vi "Find Best Merge Candidate.vi"(11 "Lines":T1[](array[typedef])) -> (0 "Best Match Outlier Distance":dbl, 2 "Best match second index":i32, 3 "Best match first index":i32)   [LabVIEW 2017]
uses:
  Vector Library/Line.ctl
  Vector Library/Vector.ctl
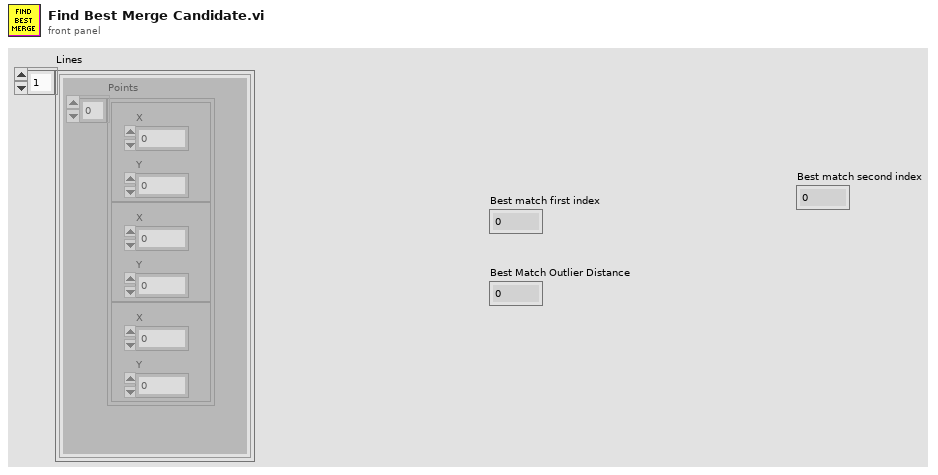
[diagram p1: front panel]
types:
  T1 = typedef "Line.ctl" = cluster{"Points":T2[]}
  T2 = typedef "Vector.ctl" = cluster{"X":dbl, "Y":dbl}
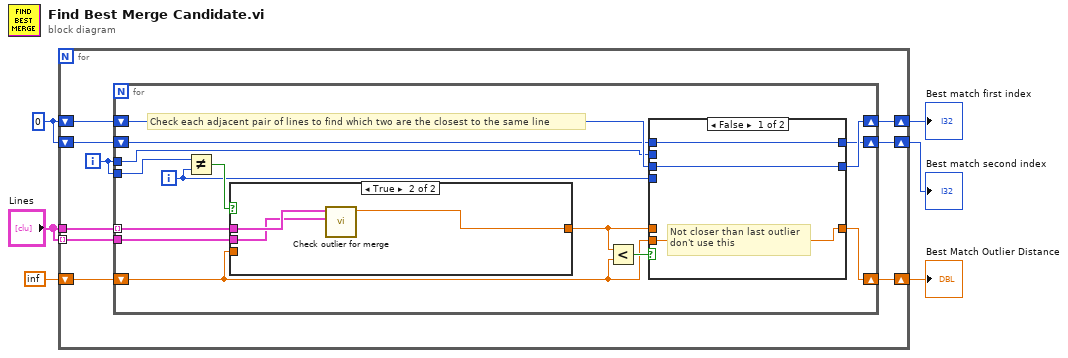
[diagram p0: block diagram]
diagram:
  w2 = 0
  n1 = for {
    tunnel: "Lines" -> [w12] mode=indexing
    shift-right: [w14] -> w5
    shift-left: inf -> [w15]
    shift-right: [w13] -> w4
    shift-left: w2 -> [w10]
    tunnel: "Lines" -> [w11]
    shift-right: [w8] -> w1
    shift-left: w2 -> [w9]
    i -> [w7]
    n2 = for {
      shift-right: [w27] -> w14
      shift-left: w15 -> [w16]
      shift-right: [w29] -> w13
      shift-left: w10 -> [w28]
      tunnel: w12 -> [w25]
      tunnel: w11 -> [w20] mode=indexing
      tunnel: w7 -> [w21]
      shift-right: [w19] -> w8
      shift-left: w9 -> [w18]
      tunnel: w7 -> [w17]
      i -> [w22]
      # "Check each adjacent pair of lines to find which two are the closest to the same line"
      n3 = Not Equal?(x=w21, y=w22) -> (x != y?=w26:bool)
      n4 = case shown="True" w26 {
        tunnel: [w30 w33] -> w24
        tunnel: w25 -> [_ w31]
        tunnel: w20 -> [_ w32]
        tunnel: w16 -> [w30 _]
        frame False {
          # "These are the same index, we don't want to compare"
        }
        frame True {
          n5 = call "Check outlier for merge.vi"("Line 2"=w31, "Line 1"=w32) -> ("Largest Outlier Distance"=w33:dbl)  [unwired: 9 in]
        }
      }
      n6 = Less?(x=w24, y=w16) -> (x < y?=w23:bool)
      n7 = case shown="False" w23 {
        tunnel: [w36 w38] -> w29
        tunnel: w28 -> [w36 _]
        tunnel: w16 -> [w35 _]
        tunnel: [w35 w39] -> w27
        tunnel: w24 -> [_ w39]
        tunnel: w22 -> [_ w38]
        tunnel: [w34 w37] -> w19
        tunnel: w18 -> [w34 _]
        tunnel: w17 -> [_ w37]
        frame False {
          # "Not closer than last outlier\ndon't use this"
        }
        frame True {
          # "Closer than best outlier\nuse this"
        }
      }
    }
  }
  "Best match first index" <- w4
  "Best Match Outlier Distance" <- w5
  "Best match second index" <- w1
